vi "Check Vectors.vi"(8 "Column":i32, 9 "Row":i32, 10 "Opponent's Tiles":bool[][](array[boolean]), 11 "Current Player's Tiles":bool[][](array[boolean])) -> (2 "Possible Flips":cluster{T1[]}[](array[cluster]), 3 "Possible Location":bool)   [LabVIEW 2020, in "Reversi.lvlib" / "Reversi.lvclass"]
uses:
  Reversi.lvclass
  Space Coordinates.ctl
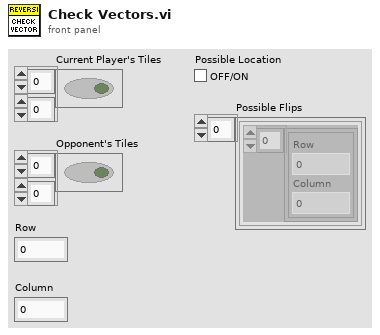
[diagram p1: front panel]
types:
  T1 = typedef "Reversi.lvlib/Reversi.lvclass/Space Coordinates.ctl" = cluster{"Row":i32, "Column":i32}
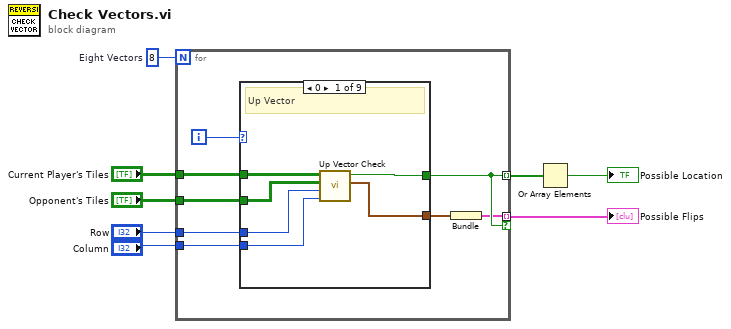
[diagram p0: block diagram]
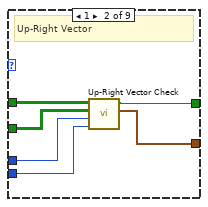
[diagram p2: hidden frame]
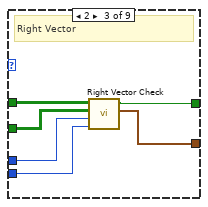
[diagram p3: hidden frame]
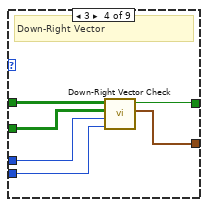
[diagram p4: hidden frame]
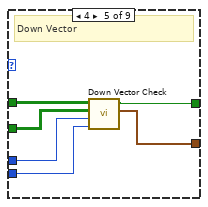
[diagram p5: hidden frame]
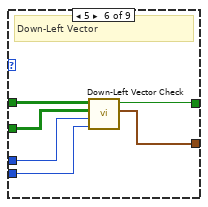
[diagram p6: hidden frame]
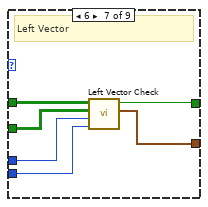
[diagram p7: hidden frame]
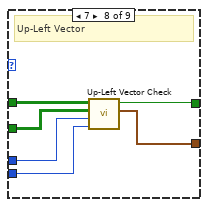
[diagram p8: hidden frame]
diagram:
  w8 = 8  # Eight Vectors
  n1 = for {
    N: w8 -> [_]
    tunnel: "Current Player's Tiles" -> [w15]
    tunnel: "Opponent's Tiles" -> [w14]
    tunnel: "Row" -> [w13]
    tunnel: "Column" -> [w12]
    tunnel: [w11] -> w3 mode=indexing
    tunnel: [w10] -> w1 mode=indexing if=w11
    i -> [w16]
    n2 = case shown="0" w16 {
      tunnel: w15 -> [w22 w27 w32 w40 w46 w52 w58 w64 _]
      tunnel: w14 -> [w21 w25 w31 w37 w43 w49 w55 w61 _]
      tunnel: w13 -> [w19 w26 w33 w38 w44 w50 w56 w62 _]
      tunnel: w12 -> [w17 w28 w34 w39 w45 w51 w57 w63 _]
      tunnel: [w20 w24 w30 w36 w42 w48 w54 w60 _] -> w11
      tunnel: [w18 w23 w29 w35 w41 w47 w53 w59 _] -> w9
      frame 0 {
        # "Up Vector"
        n3 = call "Up Vector Check.vi"("Column"=w17, "Row"=w19, "Opponent's Tiles"=w21, "Current Player's Tiles"=w22) -> ("Possible Flips"=w18:T1[], "Possible Location"=w20:bool)  [unwired: 6 in]
      }
      frame 1 {
        # "Up-Right Vector"
        n4 = call "Up-Right Vector Check.vi"("Column"=w28, "Row"=w26, "Opponent's Tiles"=w25, "Current Player's Tiles"=w27) -> ("Possible Flips"=w23:T1[], "Possible Location"=w24:bool)  [unwired: 6 in]
      }
      frame 2 {
        # "Right Vector"
        n5 = call "Right Vector Check.vi"("Column"=w34, "Row"=w33, "Opponent's Tiles"=w31, "Current Player's Tiles"=w32) -> ("Possible Flips"=w29:T1[], "Possible Location"=w30:bool)  [unwired: 6 in]
      }
      frame 3 {
        # "Down-Right Vector"
        n6 = call "Down-Right Vector Check.vi"("Column"=w39, "Row"=w38, "Opponent's Tiles"=w37, "Current Player's Tiles"=w40) -> ("Possible Flips"=w35:T1[], "Possible Location"=w36:bool)  [unwired: 6 in]
      }
      frame 4 {
        # "Down Vector"
        n7 = call "Down Vector Check.vi"("Column"=w45, "Row"=w44, "Opponent's Tiles"=w43, "Current Player's Tiles"=w46) -> ("Possible Flips"=w41:T1[], "Possible Location"=w42:bool)  [unwired: 6 in]
      }
      frame 5 {
        # "Down-Left Vector"
        n8 = call "Down-Left Vector Check.vi"("Column"=w51, "Row"=w50, "Opponent's Tiles"=w49, "Current Player's Tiles"=w52) -> ("Possible Flips"=w47:T1[], "Possible Location"=w48:bool)  [unwired: 6 in]
      }
      frame 6 {
        # "Left Vector"
        n9 = call "Left Vector Check.vi"("Column"=w57, "Row"=w56, "Opponent's Tiles"=w55, "Current Player's Tiles"=w58) -> ("Possible Flips"=w53:T1[], "Possible Location"=w54:bool)  [unwired: 6 in]
      }
      frame 7 {
        # "Up-Left Vector"
        n10 = call "Up-Left Vector Check.vi"("Column"=w63, "Row"=w62, "Opponent's Tiles"=w61, "Current Player's Tiles"=w64) -> ("Possible Flips"=w59:T1[], "Possible Location"=w60:bool)  [unwired: 6 in]
      }
      frame Default {
      }
    }
    n11 = Bundle("Possible Flips"=w9) -> (w10:cluster{"Possible Flips":T1[]})  [unwired: 1 in]
  }
  "Possible Flips" <- w1
  n12 = Or Array Elements(Boolean array=w3) -> (logical OR=→"Possible Location":bool)
